vi "INA219 Read Measurements.vi"(7 "I2C Channel":u8, 8 "error in (no error)":errorcluster, 9 "INA219 Config Options":T1={"Reset bit"=0, "Bus Voltage Range"=1, "PGA/Shunt Voltage Gain"=3, "Bus Voltage ADC Settings"=8, "Shunt Voltage ADC Settings"=3, "Mode"=7, "Calibration Value"=4096} {"Calibration Value" format="%.0x"; "Mode" items=["Power Down", "Shunt Voltage, Triggered", "Bus Voltage, Triggered", "Shunt & Bus, Triggered", "ADC Off (Disabled)", "Shunt Voltage, Continuous", "Bus Voltage, Continuous", "Shunt & Bus Voltage, Continuous"]; "Shunt Voltage ADC Settings" items=["9-bit, 84us conversion time"=0, "10-bit, 148us conversion time"=1, "11-bit, 276us conversion time"=2, "12-bit, 532us conversion time"=3, "1x12-bit, 532us conversion time"=8, "2x12-bit averaged, 1.06ms conversion time"=9, "4x12-bit averaged, 2.13ms conversion time"=10, "8x12-bit averaged, 4.26ms conversion time"=11, "16x12-bit averaged, 8.51ms conversion time"=12, "32x12-bit averaged, 17.02ms conversion time"=13, "64x12-bit averaged, 34.05ms conversion time"=14, "128x12-bit averaged, 68.10ms conversion time"=15]; "Bus Voltage ADC Settings" items=["9-bit, 84us conversion time"=0, "10-bit, 148us conversion time"=1, "11-bit, 276us conversion time"=2, "12-bit, 532us conversion time"=3, "1x12-bit, 532us conversion time"=8, "2x12-bit averaged, 1.06ms conversion time"=9, "4x12-bit averaged, 2.13ms conversion time"=10, "8x12-bit averaged, 4.26ms conversion time"=11, "16x12-bit averaged, 8.51ms conversion time"=12, "32x12-bit averaged, 17.02ms conversion time"=13, "64x12-bit averaged, 34.05ms conversion time"=14, "128x12-bit averaged, 68.10ms conversion time"=15]; "PGA/Shunt Voltage Gain" items=["Gain 1, +/-40mV", "Gain 2, +/-80mV", "Gain 3, +/-160mV", "Gain 4, +/-320mV"]; "Bus Voltage Range" items=["0-16V Range", "0-32V Range"]; "Reset bit" items=["Do Not Reset", "Reset"]}, 10 "I2C Slave Address":u8 format="%.0x", 11 "LINX Resource in":T3) -> (0 "error out":errorcluster, 2 "Measurements":T2 {"Current" format="%#.3g A"; "Power" format="%#.3g W"; "Shunt Voltage" format=" %#.3g V"; "Bus Voltage" format="%#.3g V"; "Voltage (Total)" format="%#.3g V"}, 3 "LINX Resource":T3)   [LabVIEW 2014]
uses:
  <vilib>/MakerHub/LINX/Private/Type Defs/LINX Ref.ctl
  <vilib>/MakerHub/LINX/Private/Type Defs/Platform.ctl
  <vilib>/MakerHub/LINX/Private/Type Defs/Interface.ctl
  <vilib>/MakerHub/LINX/Private/Device/Type Defs/LINX Device Config.ctl
  <vilib>/MakerHub/LINX/Private/Device/Type Defs/TCP Config.ctl
  <vilib>/MakerHub/LINX/Private/Device/Type Defs/Channels.ctl
  INA219 Measurements.ctl
  INA219 Config Options.ctl
  <vilib>/MakerHub/LINX/Private/Local IO/LinxI2cWrite.vi
  <vilib>/MakerHub/LINX/Public/Utilities/Check Channel.vi
  <vilib>/myRIO/Instrument Drivers/Onboard IO/I2C/vis/Write.vi
  <vilib>/MakerHub/LINX/Private/Utilties/Generate Error.vi
  <vilib>/MakerHub/LINX/Private/Utilties/Channel FGVs/I2C Channels.vi
  <vilib>/Utility/error.llb/Error Cluster From Error Code.vi
  <vilib>/myRIO/Common/Instrument Driver Framework/myRIO v1.0/I2C/vis/myRIO v1.0 Write I2C.vi
  <vilib>/MakerHub/LINX/LMH-LINX.lvlib
  <vilib>/MakerHub/LINX/Private/Device/Device.lvlib
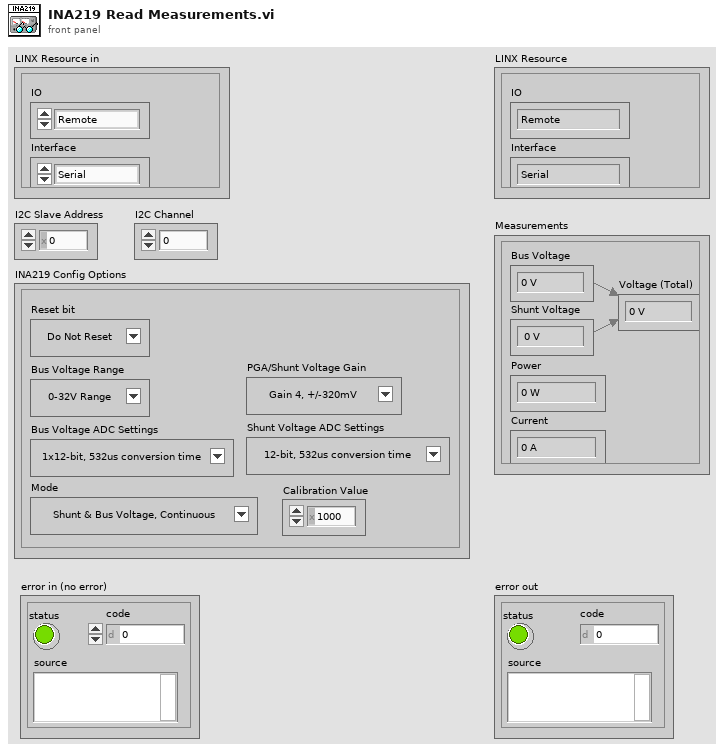
[diagram p1: front panel]
types:
  T1 = typedef "INA219 Config Options.ctl" = cluster{"Reset bit":u8, "Bus Voltage Range":u8, "PGA/Shunt Voltage Gain":u8, "Bus Voltage ADC Settings":u8, "Shunt Voltage ADC Settings":u8, "Mode":u8, "Calibration Value":u16}
  T2 = typedef "INA219 Measurements.ctl" = cluster{"Voltage (Total)":dbl, "Bus Voltage":dbl, "Shunt Voltage":dbl, "Power":dbl, "Current":dbl}
  T3 = typedef "LMH-LINX.lvlib/LINX Ref.ctl" = cluster{"IO":T4, "Interface":T5, "LINX Device Config":T6}
  T4 = typedef "LMH-LINX.lvlib/Platform.ctl" = enum16{"Remote", "Local"}
  T5 = typedef "LMH-LINX.lvlib/Interface.ctl" = enum16{"Serial", "TCP"}
  T6 = typedef "LMH-LINX.lvlib/Device.lvlib/LINX Device Config.ctl" = cluster{"Interface":T5, "COM Port":refnum<visa-resource-name>, "TCP Configuration":T7, "Device Family":u8, "Device ID":u8, "Device Name":string, "TCP Ref":refnum<k5>, "Channels":T8}
  T7 = typedef "LMH-LINX.lvlib/Device.lvlib/TCP Config.ctl" = cluster{"IP Address":string, "Port":u16}
  T8 = typedef "LMH-LINX.lvlib/Channels.ctl" = cluster{"DI":u8[], "DO":u8[], "AI":u8[], "AO":u8[], "PWM":u8[], "QE":u8[], "UART":u8[], "I2C 2":u8[], "SPI":u8[], "CAN":u8[], "Servo":u8[], "AI Ref (V)":dbl, "AI Resolution (Bits)":u8, "AO Ref (V)":dbl, "AO Resolution (Bits)":u8}
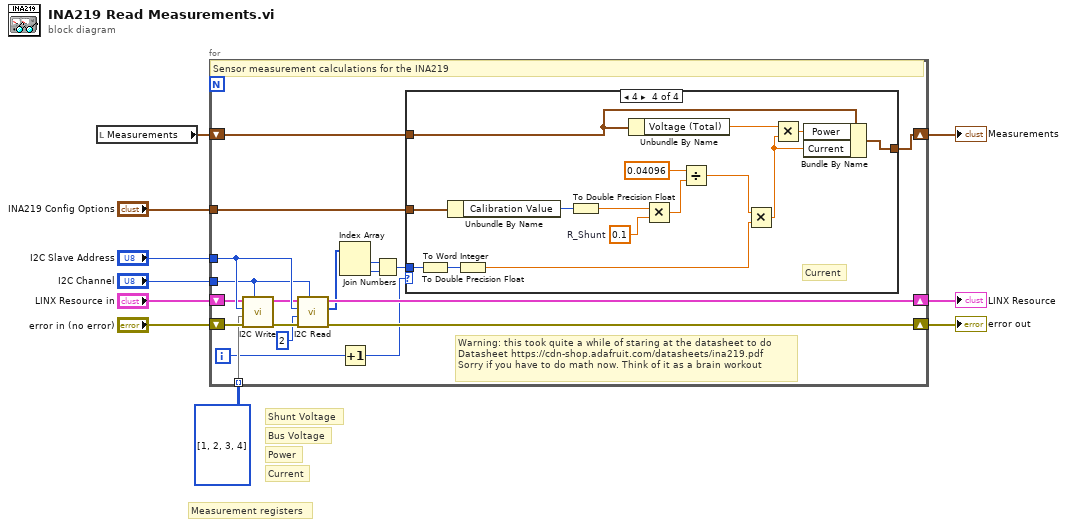
[diagram p0: block diagram]
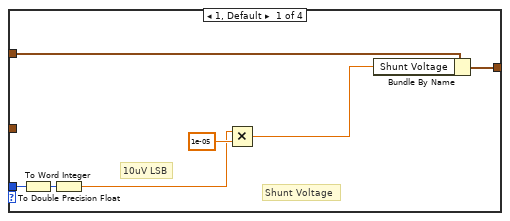
[diagram p2: hidden frame]
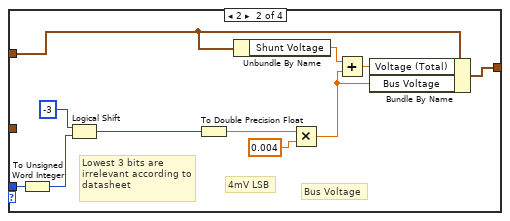
[diagram p3: hidden frame]
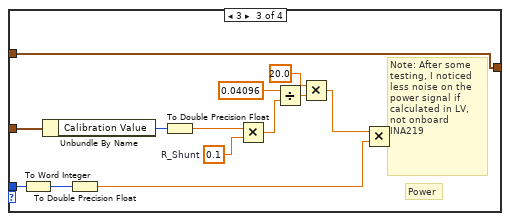
[diagram p4: hidden frame]
diagram:
  # "Measurement registers"
  # "Current"
  # "Power"
  # "Bus Voltage"
  # "Shunt Voltage"
  n1 = local read "Measurements"() -> (w3:T2)
  n2 = for {
    tunnel: "I2C Slave Address" -> [w29]
    tunnel: "I2C Channel" -> [w28]
    shift-right: [w23] -> w6
    shift-left: "error in (no error)" -> [w27]
    shift-right: [w22] -> w5
    shift-left: "LINX Resource in" -> [w26]
    tunnel: u8[][] [[1], [2], [3], [4]] ("Data") -> [w20] mode=indexing
    tunnel: "INA219 Config Options" -> [w13]
    shift-right: [w11] -> w1
    shift-left: w3 -> [w12]
    i -> [w16]
    # "Warning: this took quite a while of staring at the datasheet to do\nDatasheet https://cdn-shop.adafruit.com/datasheets/ina219.pdf\nSorry if you have to do math now. Think of it as a brain workout"
    # "Sensor measurement calculations for the INA219"
    n3 = call <vilib>:"I2C Write.vi"("I2C Channel"=w28, "Error In"=w27, "Data"=w20, "I2C Slave Address (0)"=w29, "LINX Resource"=w26) -> ("Error Out"=w24:errorcluster, "LINX Resource"=w25:T3)  [unwired: 5 in]
    n4 = call <vilib>:"I2C Read.vi"("I2C Channel"=w28, "Error In"=w24, "Bytes To Read"=u8 2, "I2C Slave Address (0)"=w29, "LINX Resource"=w25) -> ("Error Out"=w23:errorcluster, "Data"=w19:u8[], "LINX Resource"=w22:T3)  [unwired: 4 in]
    n5 = Index Array(array=w19) -> (element #1=w17:u8, element #2=w18:u8)  [unwired: 2 in]
    n6 = Increment(x=w16) -> (x+1=w15:i32)
    n7 = Join Numbers(hi=w17, lo=w18) -> ((hi.lo)=w14:u16)
    n8 = case shown="4" w15 {
      tunnel: w14 -> [w35 w41 w59 w74]
      tunnel: w13 -> [_ _ w60 w75]
      tunnel: w12 -> [w36 w46 w48 w64]
      tunnel: [w32 w47 w48 w72] -> w11
      frame 1, Default {
        # "10uV LSB"
        # "Shunt Voltage"
        n9 = To Word Integer(number=w35) -> (16bit integer=w33:i16)
        n10 = To Double Precision Float(number=w33) -> (double precision float=w30:dbl)
        n11 = Multiply(x=w30, y=1e-05) -> (x*y=w34:dbl)
        n12 = Bundle By Name(cluster=w36, "Shunt Voltage"=w34) -> (w32:T2)
      }
      frame 2 {
        # "Lowest 3 bits are irrelevant according to datasheet"
        # "4mV LSB"
        # "Bus Voltage"
        n13 = To Unsigned Word Integer(number=w41) -> (unsigned 16bit integer=w40:u16)
        n14 = Logical Shift(y=i16 -3, x=w40) -> (x << y=w38:u16)
        n15 = To Double Precision Float(number=w38) -> (double precision float=w42:dbl)
        n16 = Unbundle By Name(w46) -> ("Shunt Voltage"=w44:dbl)
        n17 = Multiply(x=w42, y=0.004) -> (x*y=w45:dbl)
        n18 = Add(x=w44, y=w45) -> (x+y=w37:dbl)
        n19 = Bundle By Name(cluster=w46, "Voltage (Total)"=w37, "Bus Voltage"=w45) -> (w47:T2)
      }
      frame 3 {
        w58 = 0.1  # R_Shunt
        # "Note: After some testing, I noticed less noise on the power signal if calculated in LV, not onboard INA219"
        # "Power"
        n20 = To Word Integer(number=w59) -> (16bit integer=w53:i16)
        n21 = Unbundle By Name(w60) -> ("Calibration Value"=w54:u16)
        n22 = To Double Precision Float(number=w53) -> (double precision float=w52:dbl)
        n23 = To Double Precision Float(number=w54) -> (double precision float=w55:dbl)
        n24 = Multiply(x=w55, y=w58) -> (x*y=w57:dbl)
        n25 = Divide(x=0.04096, y=w57) -> (x/y=w50:dbl)
        n26 = Multiply(x=20.0, y=w50) -> (x*y=w51:dbl)
        n27 = Multiply(x=w51, y=w52) -> ()  [unwired: 1 out]
      }
      frame 4 {
        w71 = 0.1  # R_Shunt
        # "Current"
        n28 = To Word Integer(number=w74) -> (16bit integer=w73:i16)
        n29 = Unbundle By Name(w75) -> ("Calibration Value"=w68:u16)
        n30 = To Double Precision Float(number=w73) -> (double precision float=w66:dbl)
        n31 = To Double Precision Float(number=w68) -> (double precision float=w67:dbl)
        n32 = Unbundle By Name(w64) -> ("Voltage (Total)"=w62:dbl)
        n33 = Multiply(x=w67, y=w71) -> (x*y=w70:dbl)
        n34 = Divide(x=0.04096, y=w70) -> (x/y=w65:dbl)
        n35 = Multiply(x=w65, y=w66) -> (x*y=w63:dbl)
        n36 = Multiply(x=w62, y=w63) -> (x*y=w61:dbl)
        n37 = Bundle By Name(cluster=w64, "Power"=w61, "Current"=w63) -> (w72:T2)
      }
    }
  }
  "error out" <- w6
  "LINX Resource" <- w5
  "Measurements" <- w1
